vi "BigAPPCreateAPI.vi"(6 "Variant in":variant, 7 "Shift Pressed?":bool, 8 "error in (no error)":errorcluster, 10 "QD Combo Box Ref":refnum<vi>, 11 "QD Launch VI Ref":refnum<vi>) -> (0 "error out":errorcluster, 4 "Variant out":variant)   [LabVIEW 2017]
doc: "Write a 1-2 sentence description of the functionality of your plugin here. Replace the \"$\" below with the character you wish to assign as the default shortcut for this plugin. Do not add any text after the 'Default Shortcut' line below.\n\nDefault Shortcut - [$]"
panel:
  in  "Undo Name":string="Quick Drop Keyboard Shortcut"
  # "Do not change the connector pane of this VI.\n\nSee the block diagram for directions on how to use this template."
  # "Specify the name of the Undo transaction"
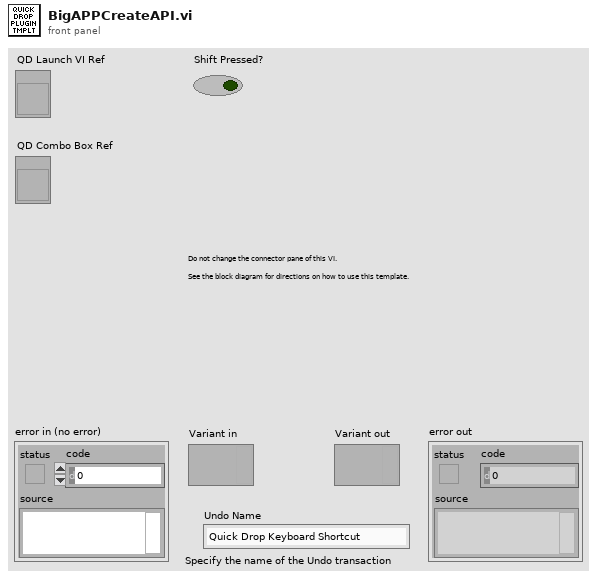
[diagram p1: front panel]
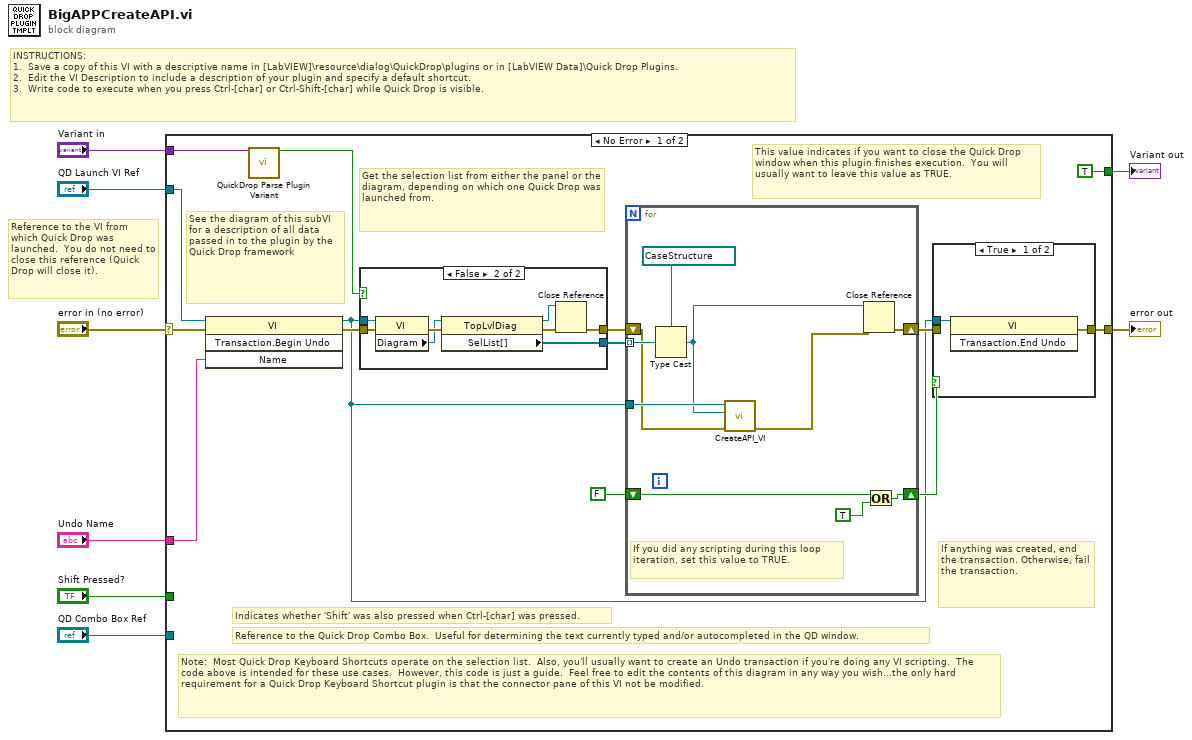
[diagram p0: block diagram]
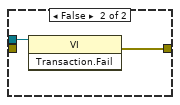
[diagram p2: hidden frame]
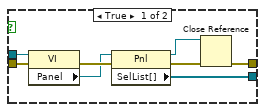
[diagram p3: hidden frame]
diagram:
  # "Reference to the VI from which Quick Drop was launched.  You do not need to close this reference (Quick Drop will close it)."
  # "INSTRUCTIONS:\n1.  Save a copy of this VI with a descriptive name in [LabVIEW]\\resource\\dialog\\QuickDrop\\plugins or in [LabVIEW Data]\\Quick Drop Plugins.\n2.  Edit the VI Description to include a description of your plugin and specify a default shortcut. \n3.  Write code to execute when you press Ctrl-[char] or Ctrl-Shift-[char] while Quick Drop is visible."
  n1 = case shown="No Error" "error in (no error)" {
    selector: "error in (no error)" -> [w21 w53]
    tunnel: [w15 w53] -> w7
    tunnel: "QD Launch VI Ref" -> [w20 _]
    tunnel: "Shift Pressed?" -> [_ _]
    tunnel: "QD Combo Box Ref" -> [_ _]
    tunnel: "Variant in" -> [w22 _]
    tunnel: "Undo Name" -> [w19 _]
    tunnel: [TRUE _] -> w1
    frame No Error {
      # "Note:  Most Quick Drop Keyboard Shortcuts operate on the selection list.  Also, you'll usually want to create an Undo transaction if you're doing any VI scripting.  The code above is intended for these use cases.  However, this code is just a guide.  Feel free to edit the contents of this diagram in any way you wish...the only hard requirement for a Quick Drop Keyboard Shortcut plugin is that the connector pane of this VI not be modified."
      # "Get the selection list from either the panel or the diagram, depending on which one Quick Drop was launched from."
      # "If anything was created, end the transaction. Otherwise, fail the transaction."
      # "This value indicates if you want to close the Quick Drop window when this plugin finishes execution.  You will usually want to leave this value as TRUE."
      # "See the diagram of this subVI for a description of all data passed in to the plugin by the Quick Drop framework"
      # "Reference to the Quick Drop Combo Box.  Useful for determining the text currently typed and/or autocompleted in the QD window."
      # "Indicates whether 'Shift' was also pressed when Ctrl-[char] was pressed."
      n2 = invoke class="VI" method="Transaction.Begin Undo"(reference=w20, error in=w21, "Name"=w19) -> (reference out=w9:refnum<vi>, error out=w16:errorcluster)  [unwired: 1 in, 2 out]
      n3 = call <vilib>:"QuickDrop Parse Plugin Variant.vi"("QDKS Variant in"=w22) -> ("QD Launch VI Panel?"=w17:bool)  [unwired: 12 in, 2 out]
      n4 = case shown="False" w17 {
        tunnel: w16 -> [w44 w52]
        tunnel: w9 -> [w43 w51]
        tunnel: [w38 w46] -> w14
        tunnel: [w37 w45] -> w10
        frame True {
          n5 = property class="VI"(reference=w43, error in=w44) -> (error out=w42:errorcluster, "Panel"=w41:refnum<vi>)  [unwired: 1 out]
          n6 = property class="Pnl"(reference=w41, error in=w42) -> (reference out=w39:refnum<vi>, error out=w40:errorcluster, "SelList[]"=w37:refnum<vi>[])
          n7 = Close Reference(reference=w39, error in (no error)=w40) -> (error out=w38:errorcluster)
        }
        frame False {
          n8 = property class="VI"(reference=w51, error in=w52) -> (error out=w50:errorcluster, "Diagram"=w49:refnum<vi>)  [unwired: 1 out]
          n9 = property class="TopLvlDiag"(reference=w49, error in=w50) -> (reference out=w47:refnum<vi>, error out=w48:errorcluster, "SelList[]"=w45:refnum<vi>[])
          n10 = Close Reference(reference=w47, error in (no error)=w48) -> (error out=w46:errorcluster)
        }
      }
      n11 = for {
        shift-right: [w29] -> w13
        shift-left: w14 -> [w23]
        shift-right: [w31] -> w11
        shift-left: FALSE -> [w32]
        tunnel: w10 -> [w28] mode=indexing
        tunnel: w9 -> [w26]
        # "If you did any scripting during this loop iteration, set this value to TRUE."
        n12 = Type Cast(type=refnum<vi> refnum ("specific class reference"), x=w28) -> (*(type *) &x=w24:refnum<vi>)
        n13 = call <resource>:"CreateAPI_VI.vi"("error in (no error)"=w23, "specific class reference"=w24, "VI Refnum"=w26) -> ("error out"=w25:errorcluster)  [unwired: 8 in]
        n14 = Close Reference(reference=w24, error in (no error)=w25) -> (error out=w29:errorcluster)
        n15 = Or(x=w32, y=TRUE ("x")) -> (x .or. y?=w31:bool)
      }
      n16 = case shown="True" w11 {
        tunnel: w9 -> [w33 w35]
        tunnel: [w34 w36] -> w15
        tunnel: w13 -> [_ _]
        frame True {
          n17 = invoke class="VI" method="Transaction.End Undo"(reference=w33) -> (error out=w34:errorcluster)  [unwired: 2 in, 2 out]
        }
        frame False {
          n18 = invoke class="VI" method="Transaction.Fail"(reference=w35) -> (error out=w36:errorcluster)  [unwired: 2 in, 2 out]
        }
      }
    }
    frame Error {
    }
  }
  "error out" <- w7
  "Variant out" <- w1
